vi "Trial 5.vi"() -> ()   [LabVIEW 2022 SP3]
uses:
  Control 10.ctl
panel:
  out "Traffic Light 2":bool[](array[boolean])
  out "Traffic 2 Color":string
  out "Traffic Light 1":bool[](array[boolean])
  in  "STOP":bool
  out "Traffic 1 Color":string
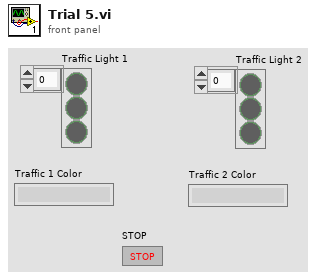
[diagram p1: front panel]
types:
  T1 = typedef "Control 10" = enum16{"Idle", "Red/Green", "Red/Amber", "Green/Red", "Amber/Red"}
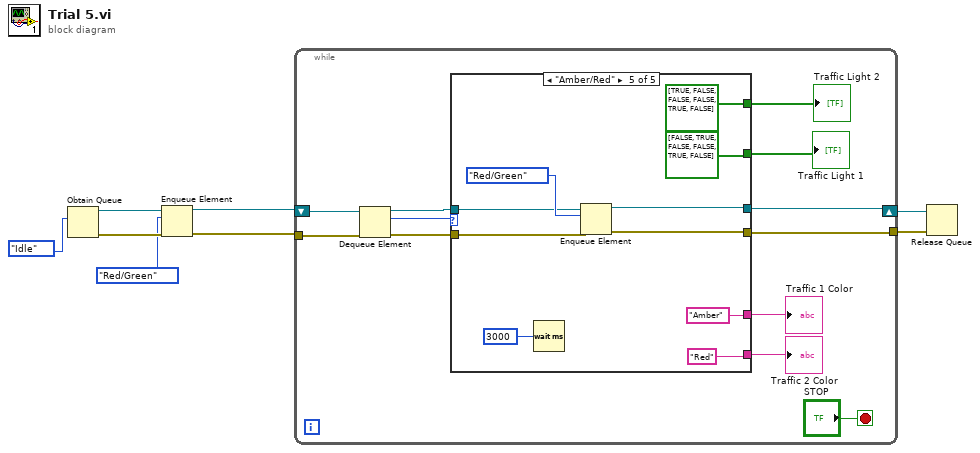
[diagram p0: block diagram]
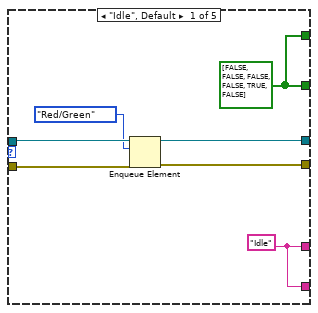
[diagram p2: hidden frame]
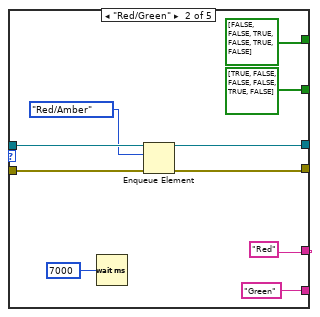
[diagram p3: hidden frame]
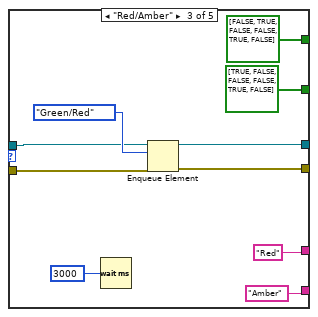
[diagram p4: hidden frame]
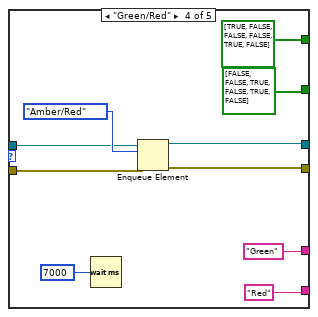
[diagram p5: hidden frame]
diagram:
  n1 = Obtain Queue(element data type=Control_10."Idle") -> (queue out=w5:refnum<queue>, error out=w4:errorcluster)  [unwired: 4 in, 1 out]
  n2 = Enqueue Element(queue=w5, element=Control_10."Red/Green", error in (no error)=w4) -> (queue out=w6:refnum<queue>, error out=w3:errorcluster)  [unwired: 1 in, 1 out]
  n3 = while {
    shift-right: [w15] -> w7
    shift-left: w6 -> [w19]
    tunnel: [w14] -> w8
    tunnel: w3 -> [w18]
    stop <- "STOP" stop-if-true
    n4 = Dequeue Element(queue=w19, error in (no error)=w18) -> (queue out=w17:refnum<queue>, element=w11:T1, error out=w16:errorcluster)  [unwired: 1 in, 1 out]
    n5 = case shown="\"Amber/Red\"" w11 {
      tunnel: w17 -> [w25 w36 w43 w55 w64]
      tunnel: w16 -> [w24 w35 w42 w54 w65]
      tunnel: [w27 w34 w41 w53 w63] -> w15
      tunnel: [w26 w33 w40 w52 w62] -> w14
      tunnel: [w22 "Red" "Red" "Green" "Amber"] -> w13
      tunnel: [w23 bool[] [TRUE, FALSE, FALSE, FALSE, TRUE, FALSE] bool[] [TRUE, FALSE, FALSE, FALSE, TRUE, FALSE] bool[] [FALSE, FALSE, TRUE, FALSE, TRUE, FALSE] bool[] [FALSE, TRUE, FALSE, FALSE, TRUE, FALSE]] -> w12
      tunnel: [w23 bool[] [FALSE, FALSE, TRUE, FALSE, TRUE, FALSE] bool[] [FALSE, TRUE, FALSE, FALSE, TRUE, FALSE] bool[] [TRUE, FALSE, FALSE, FALSE, TRUE, FALSE] bool[] [TRUE, FALSE, FALSE, FALSE, TRUE, FALSE]] -> w10
      tunnel: [w22 "Green" "Amber" "Red" "Red"] -> w9
      frame "Idle", Default {
        w23 = bool[] [FALSE, FALSE, FALSE, FALSE, TRUE, FALSE]
        w22 = "Idle"
        n6 = Enqueue Element(queue=w25, element=Control_10."Red/Green", error in (no error)=w24) -> (queue out=w27:refnum<queue>, error out=w26:errorcluster)  [unwired: 1 in, 1 out]
      }
      frame "Red/Green" {
        n7 = Wait (ms)(milliseconds to wait=7000) -> ()  [unwired: 1 out]
        n8 = Enqueue Element(queue=w36, element=Control_10."Red/Amber", error in (no error)=w35) -> (queue out=w34:refnum<queue>, error out=w33:errorcluster)  [unwired: 1 in, 1 out]
      }
      frame "Red/Amber" {
        n9 = Wait (ms)(milliseconds to wait=3000) -> ()  [unwired: 1 out]
        n10 = Enqueue Element(queue=w43, element=Control_10."Green/Red", error in (no error)=w42) -> (queue out=w41:refnum<queue>, error out=w40:errorcluster)  [unwired: 1 in, 1 out]
      }
      frame "Green/Red" {
        n11 = Wait (ms)(milliseconds to wait=7000) -> ()  [unwired: 1 out]
        n12 = Enqueue Element(queue=w55, element=Control_10."Amber/Red", error in (no error)=w54) -> (queue out=w53:refnum<queue>, error out=w52:errorcluster)  [unwired: 1 in, 1 out]
      }
      frame "Amber/Red" {
        n13 = Wait (ms)(milliseconds to wait=3000) -> ()  [unwired: 1 out]
        n14 = Enqueue Element(queue=w64, element=Control_10."Red/Green", error in (no error)=w65) -> (queue out=w63:refnum<queue>, error out=w62:errorcluster)  [unwired: 1 in, 1 out]
      }
    }
    "Traffic 1 Color" <- w13
    "Traffic Light 1" <- w12
    "Traffic Light 2" <- w10
    "Traffic 2 Color" <- w9
  }
  n15 = Release Queue(queue=w7, error in (no error)=w8) -> ()  [unwired: 1 in, 3 out]
